vi "Lift Positioner thing.vi"(11 "Operator Gamepad":T1) -> (3 "Setpoint":dbl)   [LabVIEW 2014]
uses:
  <vilib>/Rock Robotics/WPI/Joystick/WPI_JoystickDevRef.ctl
  <vilib>/Rock Robotics/WPI/Joystick/WPI_JoystickDeviceEnum.ctl
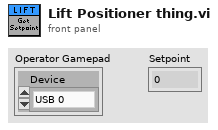
[diagram p1: front panel]
types:
  T1 = typedef "WPI_JoystickDevRef.ctl" = cluster{"Device":T2}
  T2 = typedef "WPI_JoystickDeviceEnum.ctl" = enum16{"USB 0", "USB 1", "USB 2", "USB 3", "USB 4", "USB 5"}
  T3 = cluster{"Position IN":dbl, "Position IN":dbl, "Position IN":dbl, "Position IN":dbl, "Position IN":dbl}
  T4 = cluster{"index":i32, "index":i32, "index":i32, "index":i32}
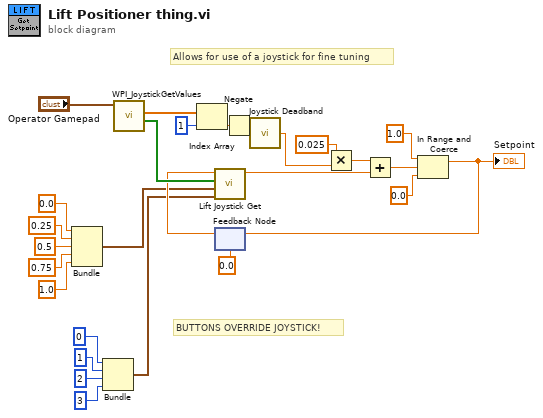
[diagram p0: block diagram]
diagram:
  # "BUTTONS OVERRIDE JOYSTICK!"
  # "Allows for use of a joystick for fine tuning"
  n1 = Bundle("Position IN"=0.0, "Position IN"=0.25, "Position IN"=0.5, "Position IN"=0.75, "Position IN"=1.0) -> (w12:T3)  [unwired: 1 in]
  n2 = Bundle("index"=0, "index"=1, "index"=2, "index"=3) -> (w6:T4)  [unwired: 1 in]
  n3 = call <vilib>:"WPI_JoystickGetValues.vi"("JoystickDevRef"="Operator Gamepad") -> ("Buttons"=w23:bool[], "Axes"=w24:dbl[])  [unwired: 6 in, 3 out]
  n4 = Index Array(array=w24, index=1) -> (element=w25:dbl)
  n5 = feedback #1(0.0 ("Position IN")) -> (w22:dbl)
  n6 = call "Lift Joystick Get.vi"("Button Index's"=w6, "Setpoints"=w12, "Joystick IN"=w23, "Position IN"=w22) -> ("Position"=w21:dbl)  [unwired: 6 in, 1 out]
  n7 = Negate(x=w25) -> (-x=w1:dbl)
  n8 = call "Joystick Deadband.vi"("Joystick Value"=w1) -> ("Joystick Output"=w17:dbl)  [unwired: 1 in]
  n9 = Multiply(x=0.025 ("Joystick Output"), y=w17) -> (x*y=w19:dbl)
  n10 = Add(x=w19, y=w21) -> (x+y=w15:dbl)
  n11 = In Range and Coerce(upper limit=1.0 ("x"), x=w15, lower limit=0.0) -> (coerced(x)=w16:dbl)  [unwired: 1 out]
  "Setpoint" <- w16
  n12 = feedback-in #1(w16) -> ()
